vi "getStopMechanism.vi"(8 "error in (no error)":errorcluster, 11 "ExampleTask_StopNotifier in":refnum<class "Task_BoolUserEventStopMech.lvclass">) -> (0 "error out":errorcluster, 2 "stopMechanism":refnum<class "ITaskStopMechanism.lvclass">, 3 "ExampleTask_StopNotifier out":refnum<class "Task_BoolUserEventStopMech.lvclass">)   [LabVIEW 2023, in "Task_BoolUserEventStopMech.lvclass"]
doc: "Returns the stop mechanism type used by the task."
uses:
  Task_BoolUserEventStopMech.lvclass
  ITaskStopMechanism/ITaskStopMechanism.lvclass
  BoolUserEventStopMech/BoolUserEventStopMechanism.lvclass
  Task_BoolUserEventStopMech.lvclass/Task_BoolUserEventStopMech.ctl
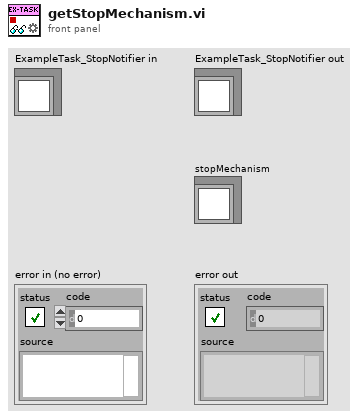
[diagram p1: front panel]
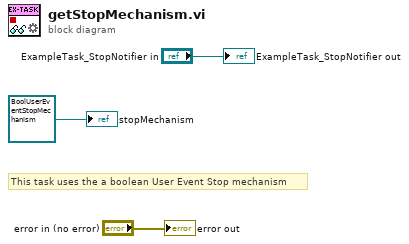
[diagram p0: block diagram]
diagram:
  # "This task uses the a boolean User Event Stop mechanism"
  "error out" <- "error in (no error)"
  "ExampleTask_StopNotifier out" <- "ExampleTask_StopNotifier in"
  "stopMechanism" <- refnum<class "BoolUserEventStopMechanism.lvclass"> refnum ("TLC_Daemon.lvlib:BoolUserEventStopMechanism.lvclass")
